vi "SysDef.Property.Get.Variant.vi"(8 "error in (no error)":errorcluster, 9 "Value":variant, 10 "Property Name":string, 11 "nodeID":u64) -> (0 "error out":errorcluster, 1 "Value":variant, 3 "nodeID out":u64, 4 "Found?":bool)   [LabVIEW 2015, in "Import - Export CD Config Utility.lvlib"]
uses:
  Import - Export CD Config Utility.lvlib
  <vilib>/NI Veristand/Custom Device API/Get Item Property (Variant).vi
  NationalInstruments.VeriStand.SystemDefinitionAPI
  <vilib>/NI Veristand/Custom Device API/Custom Device API.lvlib
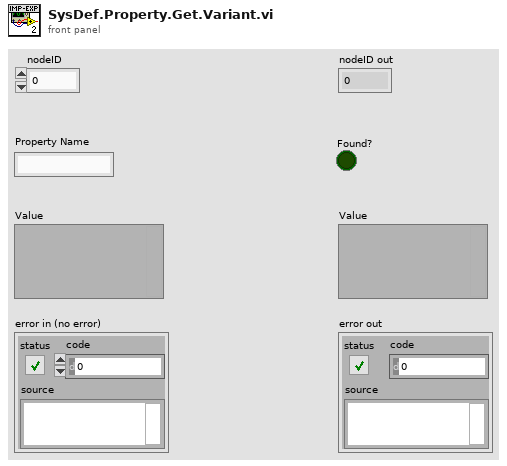
[diagram p1: front panel]
types:
  T1 = typedef "Custom Device API.lvlib/Custom Device Item Ref.ctl" = u64
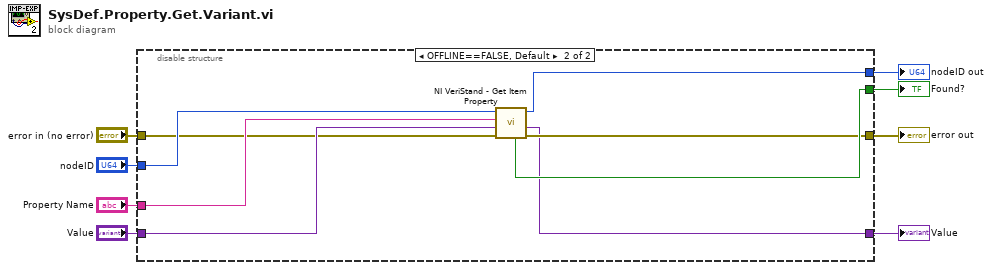
[diagram p0: block diagram]
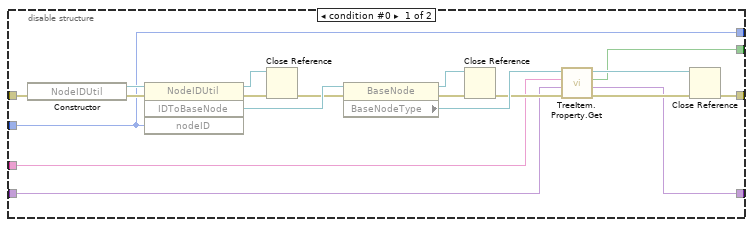
[diagram p2: hidden frame]
diagram:
  n1 = disable-structure shown="OFFLINE==FALSE, Default" {
    disable-tunnel: "error in (no error)" -> [w20 w32]
    disable-tunnel: "nodeID" -> [w11 w33]
    disable-tunnel: [w15 w30] -> w6
    disable-tunnel: "Property Name" -> [w14 w34]
    disable-tunnel: [w13 w31] -> w4
    disable-tunnel: "Value" -> [w12 w35]
    disable-tunnel: [w9 w28] -> w2
    disable-tunnel: [w11 w29] -> w1
    frame condition #0 {
      n2 = constructor class="NodeIDUtil"(error in=w20) -> (reference out=w27:refnum<k24>, error out=w26:errorcluster)  [unwired: 2 in, 1 out]
      n3 = invoke class="NodeIDUtil" method="IDToBaseNode"(reference=w27, error in=w26, "nodeID"=w11) -> (reference out=w21:refnum<k24>, error out=w23:errorcluster, "IDToBaseNode"=w25:refnum<k24>)  [unwired: 1 in, 1 out]
      n4 = Close Reference(reference=w21, error in (no error)=w23) -> (error out=w22:errorcluster)
      n5 = property class="BaseNode"(reference=w25, error in=w22) -> (reference out=w19:refnum<k24>, error out=w18:errorcluster, "BaseNodeType"=w24:refnum<k24>)
      n6 = Close Reference(reference=w19, error in (no error)=w18) -> (error out=w17:errorcluster)
      n7 = call "TreeItem.Property.Get.vi"("error in (no error)"=w17, "Default Value"=w12, "Property Name"=w14, "Basenode"=w24) -> ("error out"=w10:errorcluster, "Variant"=w9:variant, "Found?"=w13:bool, "Basenode"=w16:refnum<k24>)  [unwired: 4 in]
      n8 = Close Reference(reference=w16, error in (no error)=w10) -> (error out=w15:errorcluster)
    }
    frame condition #1 (active) {
      n9 = call-poly <vilib>:"NI VeriStand - Get Item Property.vi"("error in (no error)"=w32, "Default Value"=w35, "Property Name"=w34, "Item Ref in"=w33) -> ("error out"=w30:errorcluster, "Value"=w28:variant, "Item Ref out"=w29:T1, "Found?"=w31:bool)  [unwired: 4 in]
    }
  }
  "nodeID out" <- w1
  "error out" <- w6
  "Value" <- w2
  "Found?" <- w4
